vi "Module Init.vi"(8 "error in (no error)":errorcluster, 11 "ValveSimModule in":refnum<class "ValveSimModule.lvclass">) -> (0 "error out":errorcluster, 3 "ValveSimModule out":refnum<class "ValveSimModule.lvclass">)   [LabVIEW 2023, in "VolatusScratch.lvlib" / "ValveSimModule.lvclass"]
uses:
  ValveSimModule.lvclass
  lv-vecto/Vecto/Group DBL/Group DBL.lvclass
  Volatus/Module/Module.lvclass/Module.ctl
  VolatusConfig/VolatusConfigElement/VolatusConfigElement.lvclass/VolatusConfigElement.ctl
  ValveSimModule.lvclass/ValveSimModule.ctl
  Volatus/Module/Config.vi
  VolatusConfig/VolatusConfigElement/Element.vi
  VolatusConfig/Group/Group Config.lvclass
  VolatusConfig/Task/Task Config.lvclass
  Volatus/Module/Module.lvclass
  VolatusConfig/VolatusConfigElement/VolatusConfigElement.lvclass
  C:/dev/volatus/mts-volatus-super/libs/lv-volatus/Volatus/Module/Module.lvclass
  C:/dev/volatus/mts-volatus-super/libs/lv-volatus/VolatusScratch/ValveSimModule/ValveSimModule.lvclass
  C:/dev/volatus/mts-volatus-super/libs/lv-volatus/VolatusConfig/VolatusConfigElement/VolatusConfigElement.lvclass
  C:/dev/volatus/mts-volatus-super/libs/lv-volatus/VolatusConfig/Group/Group Config.lvclass
  C:/dev/volatus/mts-volatus-super/libs/lv-vecto/Vecto/Group/Group.lvclass
  C:/dev/volatus/mts-volatus-super/libs/lv-vecto/Vecto/Group DBL/Group DBL.lvclass
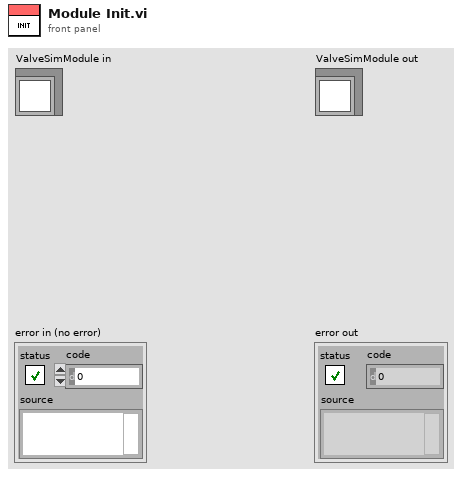
[diagram p1: front panel]
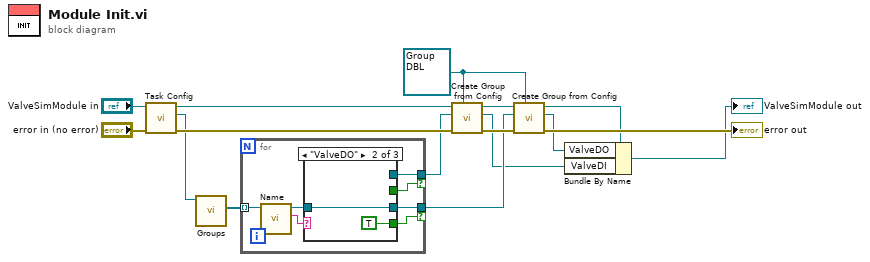
[diagram p0: block diagram]
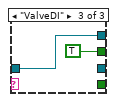
[diagram p3: hidden frame]
diagram:
  w6 = refnum<class "Group DBL.lvclass"> refnum ("ValveDI")
  n1 = call "Task Config.vi"("error in (no error)"="error in (no error)", "Module in"="ValveSimModule in") -> ("error out"=w14:errorcluster, "Task Config"=w13:refnum<class "Task Config.lvclass">, "Module out"=w10:refnum<class "ValveSimModule.lvclass">)  [unwired: 7 in]
  n2 = call "Groups.vi"("Task in"=w13) -> ("Groups"=w12:refnum<class "Group Config.lvclass">[])  [unwired: 8 in, 2 out]
  n3 = for {
    tunnel: w12 -> [w23] mode=indexing
    tunnel: [w20] -> w5 if=w19
    tunnel: [w18] -> w9 if=w17
    n4 = call "Name.vi"("VolatusConfigElement in"=w23) -> ("Name"=w22:string, "VolatusConfigElement out"=w21:refnum<class "Group Config.lvclass">)  [unwired: 8 in, 1 out]
    n5 = case shown="\"ValveDO\"" w22 {
      tunnel: w21 -> [_ w25 w27]
      tunnel: [_ w25 _] -> w20
      tunnel: [_ TRUE _] -> w19
      tunnel: [_ _ w27] -> w18
      tunnel: [_ _ TRUE] -> w17
      frame Default {
      }
      frame "ValveDO" {
      }
      frame "ValveDI" {
      }
    }
  }
  n6 = call "Create Group from Config.vi"("Group Type (Abstract)"=w6, "error in (no error)"=w14, "Group Config"=w9, "Module in"=w10) -> ("error out"=w11:errorcluster, "Group"=w3:refnum<class "Group DBL.lvclass">, "Module out"=w7:refnum<class "ValveSimModule.lvclass">)  [unwired: 5 in]
  n7 = call "Create Group from Config.vi"("Group Type (Abstract)"=w6, "error in (no error)"=w11, "Group Config"=w5, "Module in"=w7) -> ("error out"=→"error out":errorcluster, "Group"=w4:refnum<class "Group DBL.lvclass">, "Module out"=w2:refnum<class "ValveSimModule.lvclass">)  [unwired: 5 in]
  n8 = Bundle By Name(cluster=w2, "ValveDO"=w4, "ValveDI"=w3) -> (→"ValveSimModule out":refnum<class "ValveSimModule.lvclass">)
